vi "filter tags by owner.vi"(9 "exclude? (default: include)":bool, 10 "owner":string, 11 "engine configuration in":refnum<class "engine configuration.lvclass">) -> (2 "tag list":refnum<class "tag descriptor.lvclass">[](array[class]), 3 "engine configuration out":refnum<class "engine configuration.lvclass">)   [LabVIEW 2013, in "engine configuration.lvclass"]
uses:
  engine configuration.lvclass
  <vilib>/NI/Tag Bus/tag/tag descriptor.lvclass
  engine configuration.lvclass/engine configuration.ctl
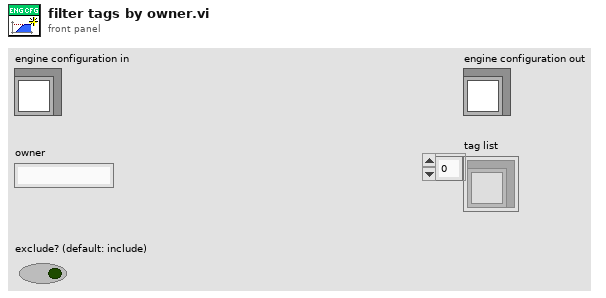
[diagram p1: front panel]
types:
  T1 = typedef "engine configuration.lvclass/Tag Info.ctl" = cluster{"Tag":refnum<class "tag descriptor.lvclass">, "Writer":string, "Readers":string[], "Owning ID":string}
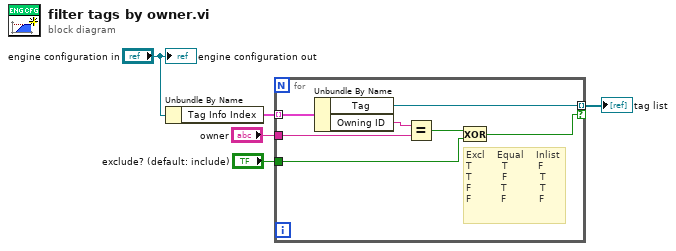
[diagram p0: block diagram]
diagram:
  n1 = Unbundle By Name("engine configuration in") -> ("Tag Info Index"=w4:T1[])
  n2 = for {
    tunnel: w4 -> [w12] mode=indexing
    tunnel: [w11] -> w3 mode=indexing if=w6
    tunnel: "exclude? (default: include)" -> [w7]
    tunnel: "owner" -> [w9]
    # "Excl    Equal    Inlist\nT          T          F \nT          F           T\nF          T           T\nF          F           F"
    n3 = Unbundle By Name(w12) -> ("Tag"=w11:refnum<class "tag descriptor.lvclass">, "Owning ID"=w10:string)
    n4 = Equal?(x=w10, y=w9) -> (x = y?=w8:bool)
    n5 = Exclusive Or(1:w7, 2:w8) -> (0:w6:bool)
  }
  "tag list" <- w3
  "engine configuration out" <- "engine configuration in"
